vi "Get Install Path From Source Path.vi"(8 "Error In":errorcluster, 10 "Source File Path":path, 11 "Configuration":T1) -> (0 "Error Out":errorcluster, 1 "Relative File Path":string, 2 "Install File Path":path, 3 "Configuration":T1)   [LabVIEW 2011, in "LVH-Build-Tools.lvlib"]
doc: "Get the install path of a file or folder from its source path.\n\nThis VI strips the source root path from the file path and prepends the install path."
uses:
  LVH-Build-Tools.lvlib
  Type Defs/Configuration.ctl
  Type Defs/Install Configuration.ctl
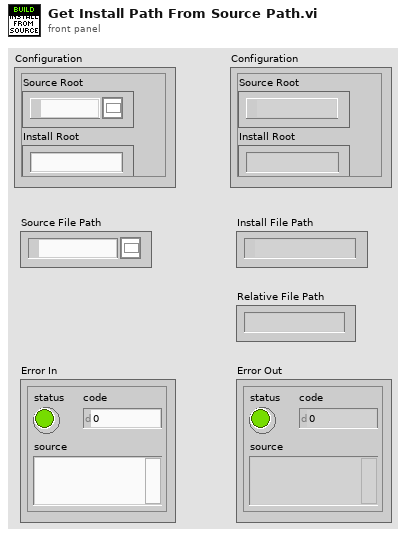
[diagram p1: front panel]
types:
  T1 = typedef "LVH-Build-Tools.lvlib/Configuration.ctl" = cluster{"Source Root":path, "Install Root":string, "Components":string[], "Ignore":string[], "Config Files":path[], "LV Directories":path[], "Install Paths":T2}
  T2 = typedef "LVH-Build-Tools.lvlib/Install Configuration.ctl" = cluster{"LabVIEW Directory":path, "Project Source Config":path}
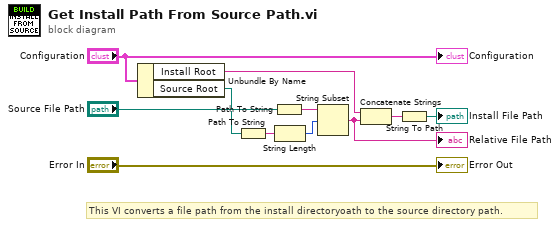
[diagram p0: block diagram]
diagram:
  # "This VI converts a file path from the install directoryoath to the source directory path."
  n1 = Unbundle By Name("Configuration") -> ("Install Root"=w4:string, "Source Root"=w2:path)
  n2 = Path To String(path=w2) -> (string=w1:string)
  n3 = Path To String(path="Source File Path") -> (string=w10:string)
  n4 = String Length(string=w1) -> (length=w11:i32)
  n5 = String Subset(string=w10, offset (0)=w11) -> (substring=w5:string)  [unwired: 1 in]
  "Relative File Path" <- w5
  n6 = Concatenate Strings(w4, w5) -> (w7:string)
  n7 = String To Path(string=w7) -> (path=→"Install File Path":path)
  "Error Out" <- "Error In"
  "Configuration" <- "Configuration"
